vi "addDeviceTree.vi"(8 "error in (no error)":errorcluster, 10 "device":string, 11 "dup tree refnum":refnum<vi>) -> (0 "error out":errorcluster, 3 "reference out":refnum<vi>)   [LabVIEW 2010]
panel:
  out "detail 2":string
  out "detail":string
  out "Edit Tree Items:Add Item":string
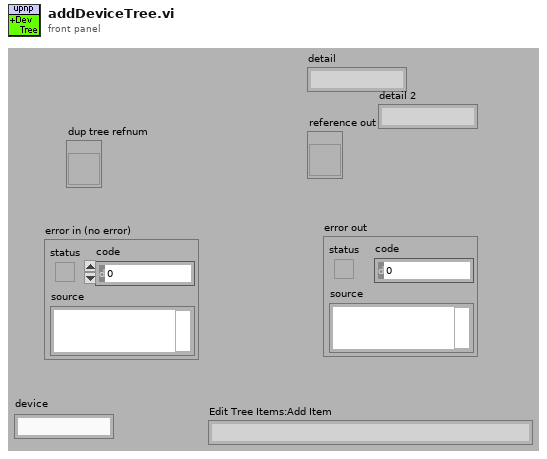
[diagram p1: front panel]
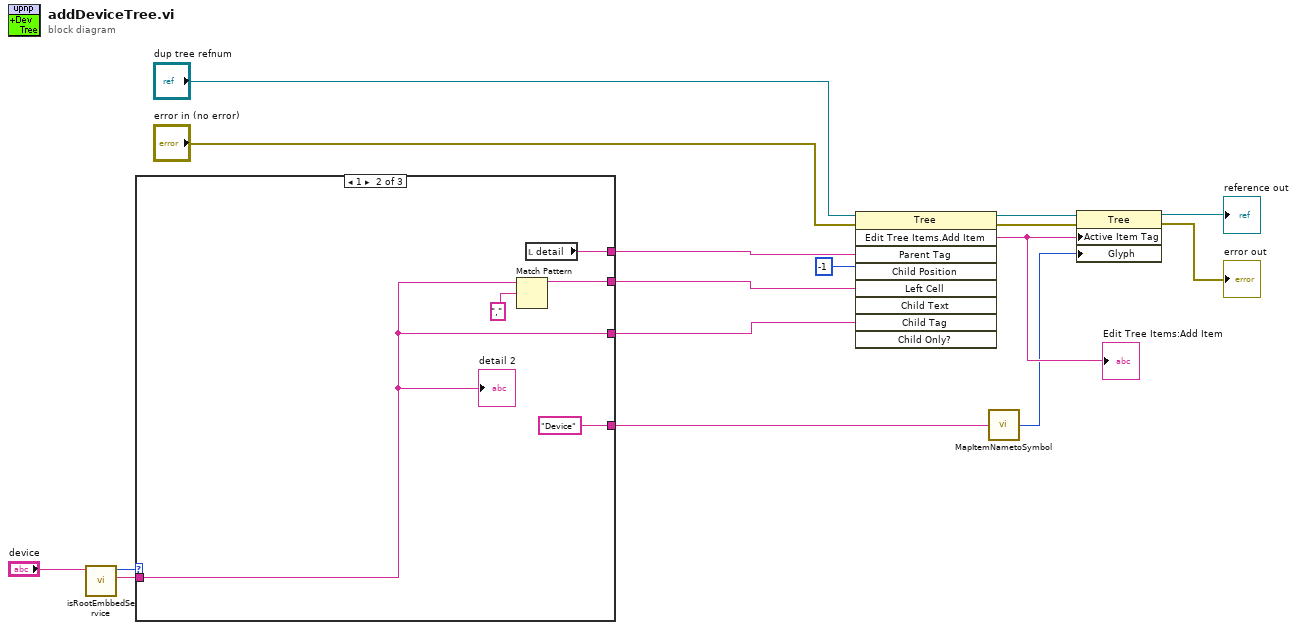
[diagram p0: block diagram]
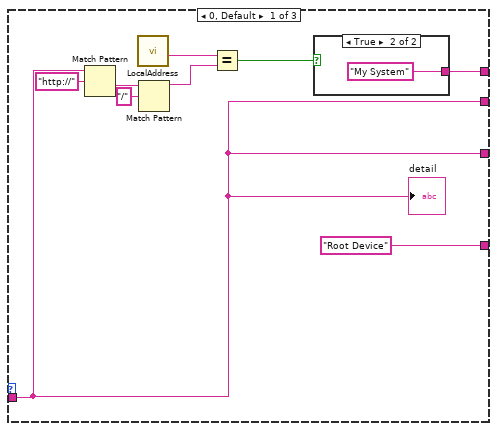
[diagram p2: hidden frame]
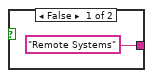
[diagram p3: hidden frame]
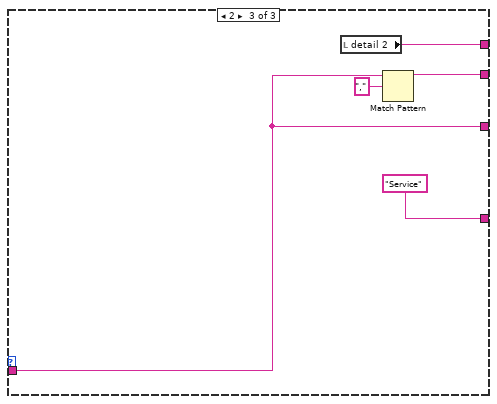
[diagram p4: hidden frame]
diagram:
  n1 = call "isRootEmbbedService.vi"("device"="device") -> ("detail"=w5:string, "type"=w15:u16)  [unwired: 9 out]
  n2 = case shown="1" w15 {
    tunnel: w5 -> [w23 w30 w35]
    tunnel: ["Root Device" "Device" "Service"] -> w4
    tunnel: [w23 w30 w35] -> w3
    tunnel: [w23 w29 w34] -> w2
    tunnel: [w17 w28 w33] -> w1
    frame 0, Default {
      n3 = Match Pattern(string=w23, regular expression="http://") -> (after substring=w21:string)  [unwired: 4 out]
      n4 = call "LocalAddress.vi"() -> ("IP Address (xx.xx.xx.xx)"=w24:string)  [unwired: 11 out]
      n5 = Match Pattern(string=w21, regular expression="/") -> (before substring=w19:string)  [unwired: 4 out]
      n6 = Equal?(x=w24, y=w19) -> (x = y?=w18:bool)
      n7 = case shown="True" w18 {
        tunnel: ["Remote Systems" ("f") "My System" ("detail 2")] -> w17
        frame False {
        }
        frame True {
        }
      }
      "detail" <- w23
    }
    frame 1 {
      n8 = Match Pattern(string=w30, regular expression=",") -> (before substring=w29:string)  [unwired: 4 out]
      n9 = local read "detail"() -> (w28:string)
      "detail 2" <- w30
    }
    frame 2 {
      n10 = local read "detail 2"() -> (w33:string)
      n11 = Match Pattern(string=w35, regular expression=",") -> (before substring=w34:string)  [unwired: 4 out]
    }
  }
  n12 = invoke class="Tree" method="Edit Tree Items.Add Item"(reference="dup tree refnum", error in="error in (no error)", "Parent Tag"=w1, "Child Position"=-1, "Left Cell"=w2, "Child Tag"=w3) -> (reference out=w11:refnum<vi>, error out=w8:errorcluster, "Edit Tree Items:Add Item"=w7:string)  [unwired: 3 in, 6 out]
  "Edit Tree Items:Add Item" <- w7
  n13 = call "MapItemNametoSymbol.vi"("Item Name"=w4) -> ("Symbol Index"=w6:i32)  [unwired: 4 out]
  n14 = property class="Tree"(reference=w11, error in=w8, "Active Item Tag"=w7, "Glyph"=w6) -> (reference out=→"reference out":refnum<vi>, error out=→"error out":errorcluster)
